vi "move-vector.vi"(5 "GetPOS Y":refnum<vi>, 7 "GetPOS X":refnum<vi>, 8 "Device in Y":refnum<k24>, 9 "X-Y":u16(ring) items=["X", "Y"], 10 "Distance":dbl, 11 "Device in X":refnum<k24>) -> (0 "Device out Y":refnum<k24>, 3 "Device out X":refnum<k24>)   [LabVIEW 2014]
doc: "André Romero - 2019\nandretec@ifsc.usp.br"
uses:
  C:/user-Lab/AndreTec/GITs/andretec/Thorlabs-Vector-Move/kinesisTec/Kinesis/Thorlabs.MotionControl.TCube.DCServoCLI.dll
  kinesisTec/Kinesis/Thorlabs.MotionControl.TCube.DCServoCLI.dll
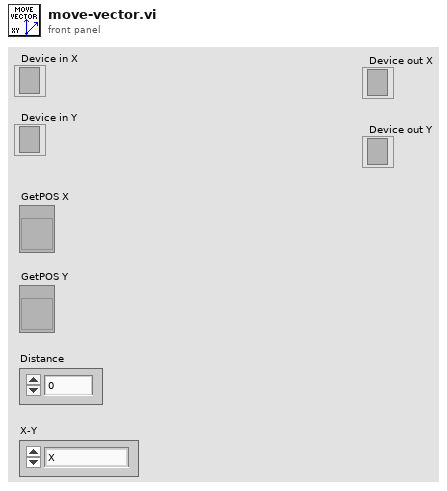
[diagram p1: front panel]
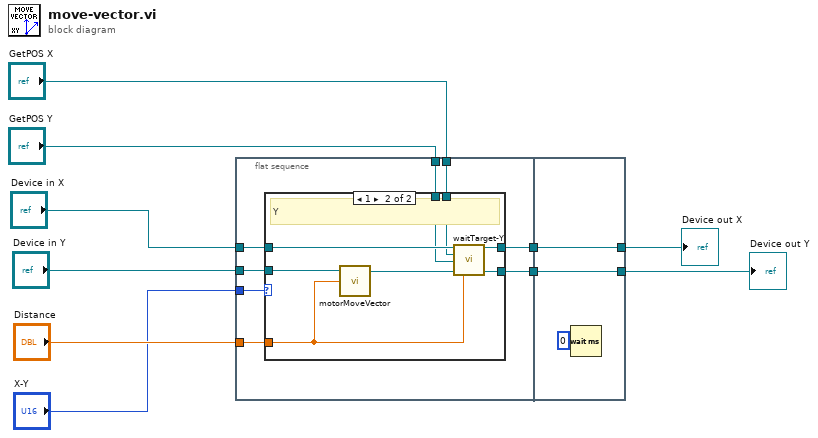
[diagram p0: block diagram]
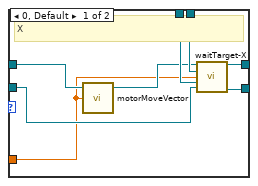
[diagram p2: hidden frame]
diagram:
  n1 = flat-sequence {
    tunnel: "Device in X" -> [w17]
    tunnel: "Device in Y" -> [w16]
    tunnel: "GetPOS Y" -> [w14]
    tunnel: "GetPOS X" -> [w13]
    tunnel: "Distance" -> [w12]
    tunnel: "X-Y" -> [w11]
    tunnel: [w18] -> w2
    tunnel: [w15] -> w1
    tunnel: [w36] -> w7
    tunnel: [w37] -> w10
    tunnel: w2 -> [w37]
    tunnel: w1 -> [w36]
    frame #0 {
      n2 = case shown="1" w11 {
        tunnel: [w23 w34] -> w18
        tunnel: w17 -> [w22 w32]
        tunnel: w16 -> [w20 w31]
        tunnel: [w24 w30] -> w15
        tunnel: w14 -> [w25 w29]
        tunnel: w13 -> [w26 w28]
        tunnel: w12 -> [w19 w27]
        frame 0, Default {
          # "X"
          n3 = call "motorMoveVector.vi"("Distance"=w19, "Device in"=w22) -> ("Device out"=w21:refnum<k24>)  [unwired: 3 in]
          n4 = call "waitTarget-X.vi"("Device in X"=w21, "GetPOS X"=w26, "Position X"=w19, "GetPOS Y"=w25, "Device in Y"=w20) -> ("Device out X"=w24:refnum<k24>, "Device out Y"=w23:refnum<k24>)  [unwired: 7 in, 2 out]
        }
        frame 1 {
          # "Y"
          n5 = call "motorMoveVector.vi"("Distance"=w27, "Device in"=w31) -> ("Device out"=w33:refnum<k24>)  [unwired: 3 in]
          n6 = call "waitTarget-Y.vi"("Device in X"=w32, "GetPOS X"=w28, "GetPOS Y"=w29, "Device in Y"=w33, "Position Y"=w27) -> ("Device out X"=w30:refnum<k24>, "Device out Y"=w34:refnum<k24>)  [unwired: 7 in, 2 out]
        }
      }
    }
    frame #1 {
      n7 = Wait (ms)(milliseconds to wait=u32 0) -> ()  [unwired: 1 out]
    }
  }
  "Device out Y" <- w10
  "Device out X" <- w7
